vi "__List Drag Enter Handler.vi"(8 "error in (no error)":errorcluster, 10 "Available data names":string[](array[string]), 11 "MCListbox Refnum":refnum<vi>) -> (0 "error out":errorcluster, 3 "Accept?":bool)   [LabVIEW 2011]
doc: "This VI decides whether a drag operation is accepted.\nIt accepts a drag operation when it enters the bound of one of the multicolumn listboxes (cloud list or local list), while the source of the operation is the opposite listbox.\nBasically it allows dragging from Local list to Cloud list or Cloud list to Local list."
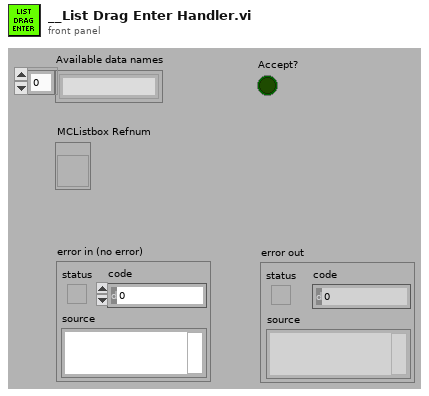
[diagram p1: front panel]
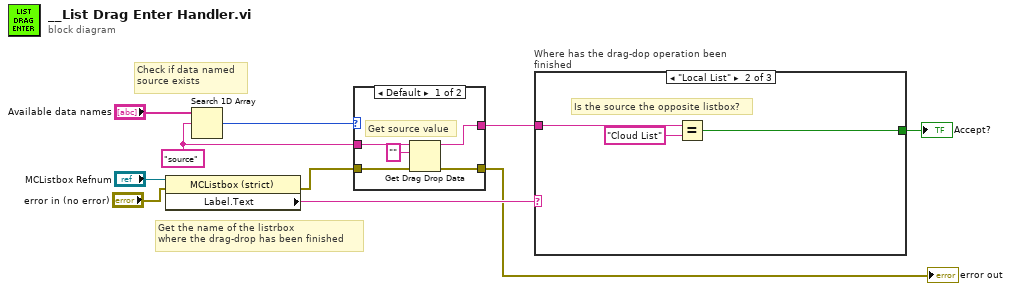
[diagram p0: block diagram]
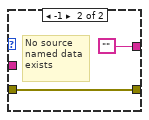
[diagram p2: hidden frame]
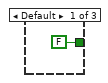
[diagram p3: hidden frame]
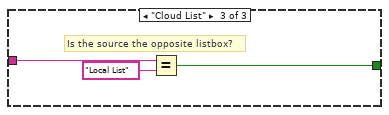
[diagram p4: hidden frame]
diagram:
  w4 = "source"
  # "Get the name of the listrbox\nwhere the drag-drop has been finished"
  # "Check if data named\nsource exists"
  n1 = property class="MCListbox (strict)"(reference="MCListbox Refnum", error in="error in (no error)") -> (error out=w3:errorcluster, "Label.Text"=w7:string)  [unwired: 1 out]
  n2 = Search 1D Array(1D array="Available data names", element=w4) -> (index of element=w5:i32)  [unwired: 1 in]
  n3 = case shown="Default" w5 {
    tunnel: w3 -> [w15 w17]
    tunnel: w4 -> [w14 _]
    tunnel: [w13 w17] -> w2
    tunnel: [w12 ""] -> w1
    frame Default {
      # "Get source value"
      n4 = Get Drag Drop Data(6:w15, 8:"" ("type"), 9:w14) -> (0:w13:errorcluster, 3:w12:string)
    }
    frame -1 {
      # "No source\nnamed data\nexists"
    }
  }
  "error out" <- w2
  n5 = case "Where has the drag-dop operation been finished" shown="\"Local List\"" w7 {
    tunnel: w1 -> [_ w21 w24]
    tunnel: [FALSE w19 w22] -> w6
    frame Default {
    }
    frame "Local List" {
      # "Is the source the opposite listbox?"
      n6 = Equal?(x=w21, y="Cloud List") -> (x = y?=w19:bool)
    }
    frame "Cloud List" {
      # "Is the source the opposite listbox?"
      n7 = Equal?(x=w24, y="Local List") -> (x = y?=w22:bool)
    }
  }
  "Accept?" <- w6
